vi "CMI ADS127L21 - Get Record Status.vi"(8 "error in (no error)":errorcluster, 11 "session in":T1 {"channels"."Channel" min=1 max=8 step=1}) -> (0 "error out":errorcluster, 1 "samples to read":i32, 2 "samples acquired":i32, 3 "session out":T1 {"channels"."Channel" min=1 max=8 step=1}, 4 "FIFO overflow?":bool, 5 "FIFO usage [%]":dbl, 6 "sampling error":bool, 7 "record running?":bool)   [LabVIEW 2020]
doc: "Get state of current record."
uses:
  CMI ADS127L21 - Session.ctl
  CMI ADS127L21 - Record Channel.ctl
  CMI ADS127L21 - Input Range.ctl
  CMI ADS127L21 - Input Mode.ctl
  CMI ADS127L21 - Input Impedance.ctl
  CMI ADS127L21 - EXTOUT Mode.ctl
  CMI ADS127L21 - EXTOUT Polarity.ctl
  <vilib>/Instr/_visa.llb/VISA Flush IO Buffer Mask.ctl
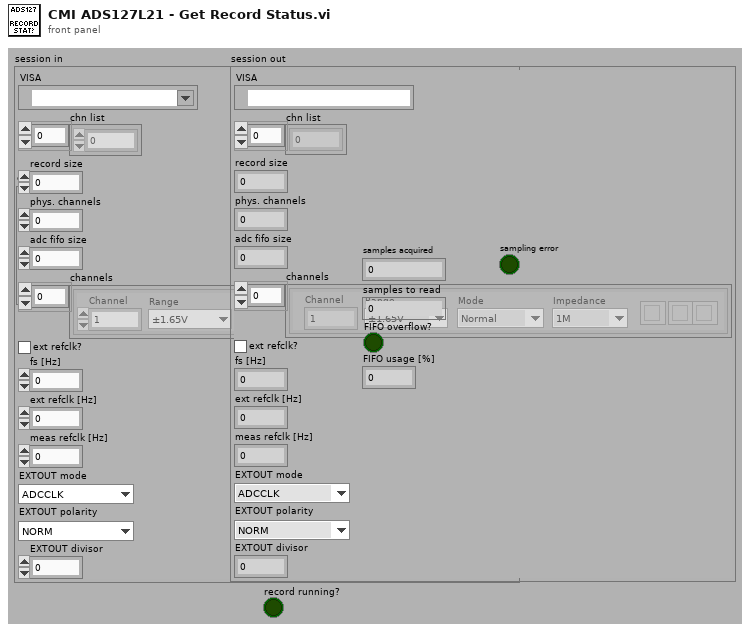
[diagram p1: front panel]
types:
  T1 = typedef "CMI ADS127L21 - Session.ctl" = cluster{"VISA":refnum<visa-resource-name>, "chn list":i32[], "record size":i32, "phys. channels":i32, "adc fifo size":i32, "channels":T2[], "ext refclk?":bool, "fs [Hz]":dbl, "ext refclk [Hz]":dbl, "meas refclk [Hz]":dbl, "EXTOUT mode":T6, "EXTOUT polarity":T7, "EXTOUT divisor":i32}
  T2 = typedef "CMI ADS127L21 - Record Channel.ctl" = cluster{"Range":T3, "Channel":i32, "Mode":T4, "Impedance":T5, "btn clr":bool, "btn up":bool, "btn down":bool}
  T3 = typedef "CMI ADS127L21 - Input Range.ctl" = enum16{"±1.65V", "±2V"}
  T4 = typedef "CMI ADS127L21 - Input Mode.ctl" = enum16{"Normal", "Inverted", "GND"}
  T5 = typedef "CMI ADS127L21 - Input Impedance.ctl" = enum16{"1M", "1k5"}
  T6 = typedef "CMI ADS127L21 - EXTOUT Mode.ctl" = enum16{"ADCCLK", "REFCLK", "SMPLCLK", "FIRST"}
  T7 = typedef "CMI ADS127L21 - EXTOUT Polarity.ctl" = enum16{"NORM", "INV"}
  T8 = enum16{"big-endian, network order", "native, host order", "little-endian"}
  T9 = typedef "VISA Flush IO Buffer Mask.ctl" = u16
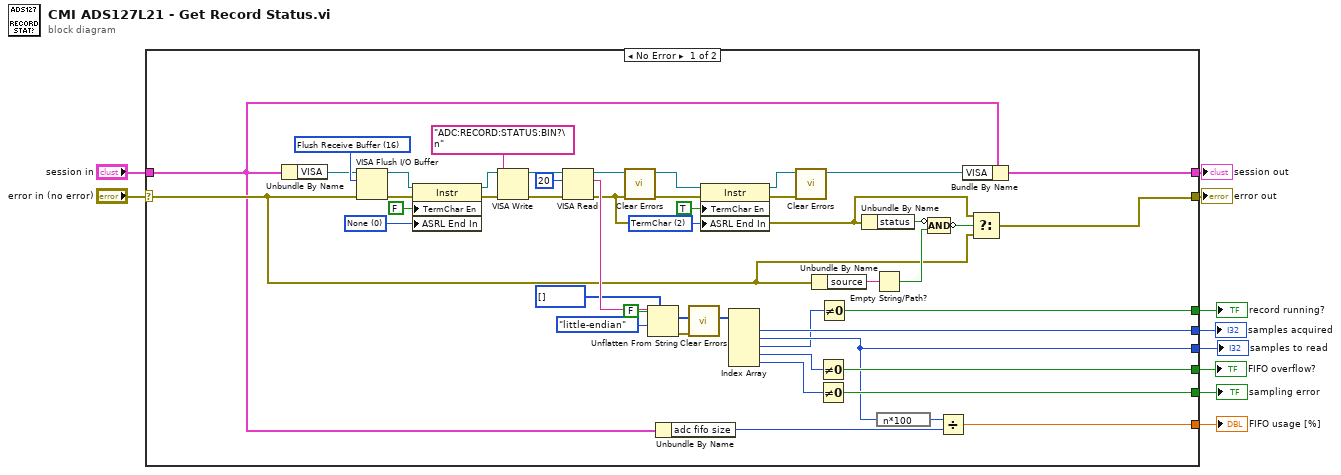
[diagram p0: block diagram]
diagram:
  n1 = case shown="No Error" "error in (no error)" {
    selector: "error in (no error)" -> [w25 w56]
    tunnel: "session in" -> [w19 w55]
    tunnel: [w53 w55] -> w9
    tunnel: [w22 w56] -> w8
    tunnel: [w40 _] -> w6
    tunnel: [w18 _] -> w5
    tunnel: [w39 _] -> w4
    tunnel: [w38 _] -> w3
    tunnel: [w15 _] -> w2
    tunnel: [w11 _] -> w1
    frame No Error {
      w26 = u16 2 items=["None", "Last Bit", "TermChar"] ("Serial Settings:End Mode for Reads")
      w27 = u16 0 items=["None", "Last Bit", "TermChar"] ("Serial Settings:End Mode for Reads")
      w52 = T9 16 items=["Flush Receive Buffer"=16, "Write Transmit Buffer to Device"=32, "Flush Receive Buffer (No I/O)"=64, "Flush Transmit Buffer"=128] ("Mask")
      n2 = Unbundle By Name(w19) -> ("VISA"=w50:refnum<visa-resource-name>)
      n3 = VISA Flush I/O Buffer(VISA resource name=w50, mask (16)=w52, error in (no error)=w25) -> (VISA resource name out=w51:refnum<visa-resource-name>, error out=w24:errorcluster)
      n4 = property class="Instr"(reference=w51, error in=w24, "TermChar En"=FALSE ("Message Based Settings:Termination Character Enable"), "ASRL End In"=w27) -> (reference out=w30:refnum<visa-resource-name>, error out=w23:errorcluster)
      n5 = VISA Write(VISA resource name=w30, write buffer="ADC:RECORD:STATUS:BIN?\n" ("format string"), error in (no error)=w23) -> (VISA resource name out=w49:refnum<visa-resource-name>, error out=w21:errorcluster)  [unwired: 1 out]
      n6 = VISA Read(VISA resource name=w49, byte count=u32 20, error in (no error)=w21) -> (VISA resource name out=w47:refnum<visa-resource-name>, read buffer=w36:string, error out=w20:errorcluster)  [unwired: 1 out]
      n7 = call <vilib>:"Clear Errors.vi"("error in (no error)"=w20) -> ("error out"=w37:errorcluster)  [unwired: 5 in, 1 out]
      n8 = Unflatten From String(type=i32[] [], binary string=w36, data includes array or string size? (T)=FALSE, byte order (0:big-endian, network order)=T8."little-endian") -> (value=w33:i32[], error out=w32:errorcluster)  [unwired: 1 in, 1 out]
      n9 = Unbundle By Name(w19) -> ("adc fifo size"=w17:i32)
      n10 = call <vilib>:"Clear Errors.vi"("error in (no error)"=w32) -> ()  [unwired: 5 in, 2 out]
      n11 = property class="Instr"(reference=w47, error in=w37, "TermChar En"=TRUE ("Message Based Settings:Termination Character Enable"), "ASRL End In"=w26) -> (reference out=w46:refnum<visa-resource-name>, error out=w41:errorcluster)
      n12 = Index Array(array=w33) -> (element #1=w40:i32, element #2=w18:i32, element #3=w12:i32, element #4=w13:i32, element #5=w14:i32)  [unwired: 5 in]
      n13 = call <vilib>:"Clear Errors.vi"("error in (no error)"=w41) -> ()  [unwired: 5 in, 2 out]
      n14 = Unbundle By Name(w25) -> ("source"=w45:string)
      n15 = Not Equal To 0?(x=w13) -> (x != 0?=w39:bool)
      n16 = Not Equal To 0?(x=w14) -> (x != 0?=w38:bool)
      n17 = Not Equal To 0?(x=w12) -> (x != 0?=w11:bool)
      n18 = Unbundle By Name(w20) -> ("status"=w44:bool)
      n19 = Empty String/Path?(string/path=w45) -> (empty?=w43:bool)
      n20 = expression code="n*100"(w18) -> (w16:i32)
      n21 = Compound Arithmetic op=AND(invert w44, w43) -> (invert w42:bool)
      n22 = Divide(x=w16, y=w17) -> (x/y=w15:dbl)
      n23 = Bundle By Name(cluster=w19, "VISA"=w46) -> (w53:T1)
      n24 = Select(t=w20, s=w42, f=w25) -> (s? t:f=w22:errorcluster)
    }
    frame Error {
    }
  }
  "error out" <- w8
  "session out" <- w9
  "samples acquired" <- w6
  "samples to read" <- w5
  "FIFO overflow?" <- w4
  "sampling error" <- w3
  "FIFO usage [%]" <- w2
  "record running?" <- w1
